vi "Receive Messages using Interrupts.vi"() -> ()   [LabVIEW 2019]
doc: "This program opens the specified card, configures the first receive channel from the configuration file with filters set for 2 messages and a default filter. The user event is created and used for reading messages received from the bus. Everytime an event log occurs, the interrupt will trigger the user event to read messages received from the bus."
uses:
  <instrlib>/BTICardLib/Private/Initialize By Card Number and Core Number.vi
  <instrlib>/BTICardLib/Private/Configure Core From XML.vi
  <instrlib>/BTI429Lib/Private/Rx/Configure/Configure Rx Channel From XML.vi
  <instrlib>/BTI429Lib/Private/Rx/Configure/Get Rx Label Handle Name.vi
  <instrlib>/BTI429Lib/Private/Core/Action-Status/Start Channel.vi
  <instrlib>/BTI429Lib/Private/Core/Action-Status/Stop Channel.vi
  <instrlib>/BTICardLib/BTICardLV.lvlib
  <instrlib>/BTI429Lib/BTI429LV.lvlib
panel:
  out "Data 2":u32 format="%x"
  out "Data 1":u32 format="%x"
  out "Default":u32 format="%x"
  out "Event Time":u32
  in  "Event Name":string="Event"
  out "rx channel number":i32
  out "core number":i32=1
  out "Error":errorcluster
  in  "Channel Configuration XML file name":string="Channel Config.xml"
  in  "Core Configuration XML file name":string="Core Config.xml"
  in  "Card Number":i32
  in  "stop":bool
  # "ARINC 429: Receive Messages using Interrupts"
  # "©2016 Astronics Ballard Technology"
  # "This program opens the specified card, configures the first receive channel from the configuration file with filters set for 2 messages and a default filter. The user event is created and used for reading messages received from the bus. Everytime an event log occurs, the interrupt will trigger the user event to read messages received from the bus."
  # "This labels for Data 1 and Data 2\nare defined in the Channel XML\nConfiguration. Shipping defaults\nare Label 206 and 211."
  # "Always Stop the card\nand Close the card when\ndone. Otherwise, the hardware\ncontinues to operate."
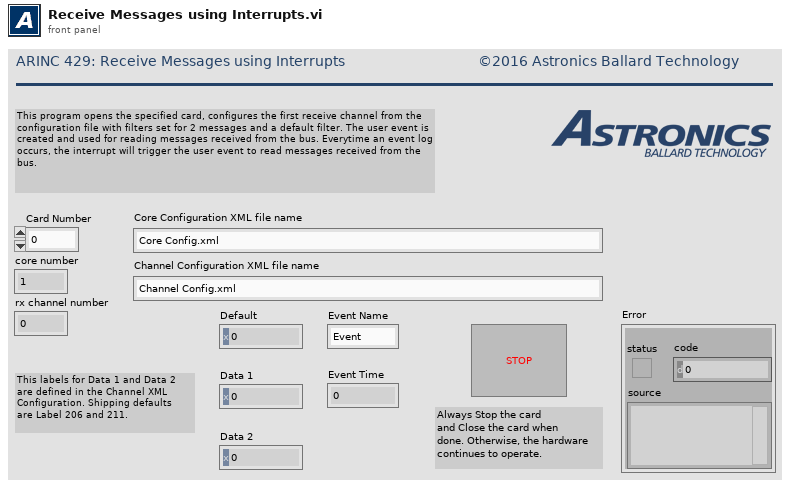
[diagram p1: front panel]
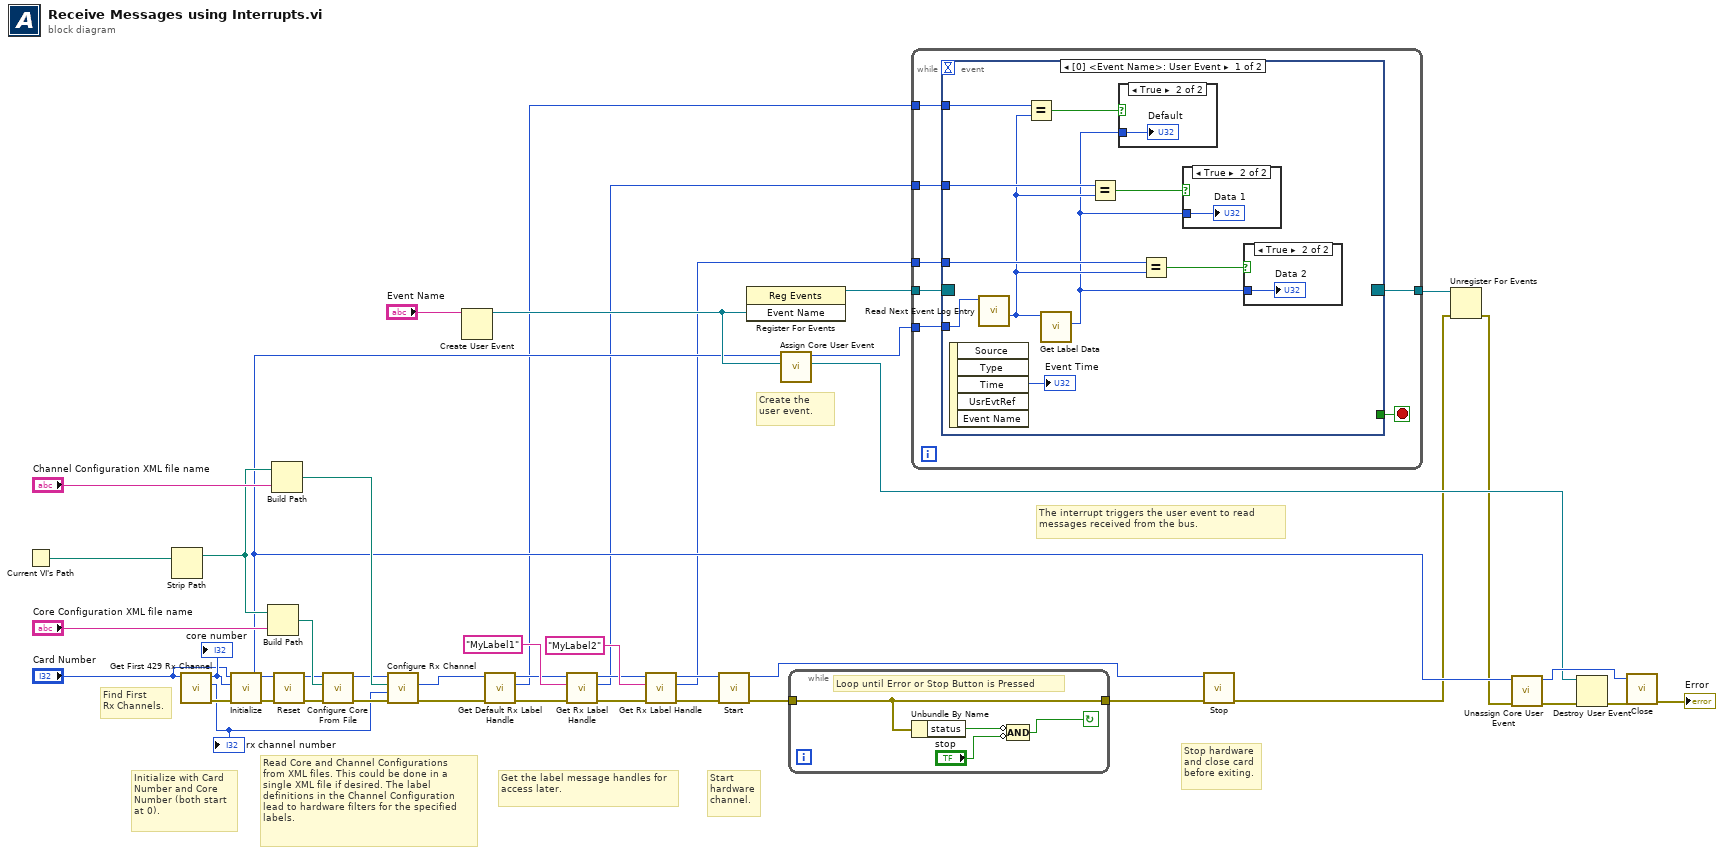
[diagram p0: block diagram]
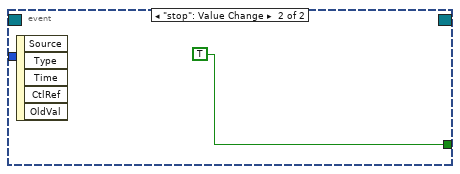
[diagram p5: hidden frame]
diagram:
  # "The interrupt triggers the user event to read messages received from the bus."
  # "Create the user event."
  # "Find First  \nRx Channels."
  # "Stop hardware\nand close card\nbefore exiting."
  # "Start\nhardware\nchannel."
  # "Get the label message handles for access later."
  # "Read Core and Channel Configurations\nfrom XML files. This could be done in a\nsingle XML file if desired. The label \ndefinitions in the Channel Configuration\nlead to hardware filters for the specified\nlabels."
  # "Initialize with Card\nNumber and Core\nNumber (both start\nat 0)."
  n1 = Current VI's Path() -> (path=w32:path)
  n2 = Strip Path(path=w32) -> (stripped path=w29:path)  [unwired: 1 out]
  n3 = call "Get First 429 Rx Channel.vi"("Card Number"="Card Number") -> ("error out"=w22:errorcluster, "Channel Number"=w19:i32, "Core Number"=w21:i32)  [unwired: 8 in]
  "core number" <- w21
  "rx channel number" <- w19
  n4 = call-poly <instrlib>:"Initialize.vi"("error in (no error)"=w22, "core number"=w21, "card number"="Card Number") -> ("error out"=w23:errorcluster, "core handle out"=w26:u64)  [unwired: 7 in]
  n5 = Build Path(base path=w29, name or relative path="Core Configuration XML file name") -> (appended path=w27:path)
  n6 = Build Path(base path=w29, name or relative path="Channel Configuration XML file name") -> (appended path=w30:path)
  n7 = call <instrlib>:"Reset.vi"("error in (no error)"=w23, "core handle in"=w26) -> ("error out"=w24:errorcluster, "core handle out"=w25:u64)  [unwired: 8 in]
  n8 = call-poly <instrlib>:"Configure Core From File.vi"("error in (no error)"=w24, "configuration file path"=w27, "core handle in"=w25) -> ("error out"=w37:errorcluster, "core handle out"=w11:u64)  [unwired: 7 in]
  n9 = call-poly <instrlib>:"Configure Rx Channel.vi"("error in (no error)"=w37, "channel number in"=w19, "configuration file path"=w30, "core handle in"=w11) -> ("error out"=w44:errorcluster, "channel handle out"=w39:u64)  [unwired: 5 in, 1 out]
  n10 = Create User Event(user event datatype="Event Name") -> (user event=w15:refnum<user-event>)  [unwired: 1 in, 1 out]
  n11 = call <instrlib>:"Get Default Rx Label Handle.vi"("error in (no error)"=w44, "channel handle in"=w39) -> ("error out"=w43:errorcluster, "default label handle out"=w7:u64, "channel handle out"=w10:u64)  [unwired: 7 in]
  n12 = call-poly <instrlib>:"Get Rx Label Handle.vi"("error in (no error)"=w43, "label name"="MyLabel1", "channel handle in"=w10) -> ("error out"=w42:errorcluster, "label handle out"=w6:u64, "channel handle out"=w9:u64)  [unwired: 6 in]
  n13 = call-poly <instrlib>:"Get Rx Label Handle.vi"("error in (no error)"=w42, "label name"="MyLabel2", "channel handle in"=w9) -> ("error out"=w41:errorcluster, "label handle out"=w5:u64, "channel handle out"=w8:u64)  [unwired: 6 in]
  n14 = call-poly <instrlib>:"Start.vi"("error in (no error)"=w41, "channel handle in"=w8) -> ("error out"=w40:errorcluster, "channel handle out"=w38:u64)  [unwired: 8 in]
  n15 = register-events(w15) -> (reference out=w17:refnum<event-registration>)  [unwired: 2 in, 1 out]
  n16 = call <instrlib>:"Assign Core User Event.vi"("user event in"=w15, "core handle in"=w11) -> ("user event out"=w12:refnum<user-event>, "core handle out"=w1:u64)  [unwired: 7 in, 1 out]
  n17 = while {
    tunnel: w40 -> [w45]
    tunnel: [w45] -> w33
    stop <- w47 continue-if-true
    # "Loop until Error or Stop Button is Pressed"
    n18 = Unbundle By Name(w45) -> ("status"=w48:bool)
    n19 = Compound Arithmetic op=AND(invert w48, invert "stop") -> (w47:bool)
  }
  n20 = while {
    tunnel: w17 -> [w55]
    tunnel: [w54] -> w16
    tunnel: w7 -> [w52]
    tunnel: w6 -> [w51]
    tunnel: w5 -> [w50]
    tunnel: w1 -> [w49]
    stop <- w53 stop-if-true
    n21 = event shown="[0] <Event Name>: User Event" {
      selector: w55 -> [_ _]
      dyn-events: [_ _] -> w54
      timeout: _ -> [_ _]
      tunnel: [_ TRUE] -> w53
      tunnel: w52 -> [w63 _]
      tunnel: w51 -> [w60 _]
      tunnel: w50 -> [w58 _]
      tunnel: w49 -> [w64 _]
      event User Event {
        n22 = event-data() -> ("Time"=→"Event Time":u32)  [unwired: 1 in, 4 out]
        n23 = call <instrlib>:"Read Next Event Log Entry.vi"("core handle in"=w64) -> ("info tag"=w57:u64)  [unwired: 5 in, 5 out]
        n24 = Equal?(x=w63, y=w57) -> (x = y?=w62:bool)
        n25 = call <instrlib>:"Get Label Data.vi"("label handle in"=w57) -> ("value"=w56:u32)  [unwired: 8 in, 2 out]
        n26 = Equal?(x=w60, y=w57) -> (x = y?=w61:bool)
        n27 = case shown="True" w62 {
          tunnel: w56 -> [_ w68]
          frame False {
          }
          frame True {
            "Default" <- w68
          }
        }
        n28 = Equal?(x=w58, y=w57) -> (x = y?=w59:bool)
        n29 = case shown="True" w61 {
          tunnel: w56 -> [_ w67]
          frame False {
          }
          frame True {
            "Data 1" <- w67
          }
        }
        n30 = case shown="True" w59 {
          tunnel: w56 -> [_ w66]
          frame False {
          }
          frame True {
            "Data 2" <- w66
          }
        }
      }
      event "stop": Value Change {
        n31 = event-data() -> ()  [unwired: 1 in, 5 out]
      }
    }
  }
  n32 = call-poly <instrlib>:"Stop.vi"("error in (no error)"=w33, "channel handle in"=w38) -> ("error out"=w4:errorcluster)  [unwired: 8 in, 1 out]
  n33 = Unregister For Events(event registration refnum=w16, error in=w4) -> (error out=w3:errorcluster)
  n34 = call <instrlib>:"Unassign Core User Event.vi"("error in (no error)"=w3, "core handle in"=w11) -> ("error out"=w2:errorcluster, "core handle out"=w14:u64)  [unwired: 8 in]
  n35 = Destroy User Event(user event=w12, error in=w2) -> (error out=w13:errorcluster)
  n36 = call <instrlib>:"Close.vi"("error in (no error)"=w13, "core handle in"=w14) -> ("error out"=→"Error":errorcluster)  [unwired: 8 in, 1 out]
